vi "Get PDOMapping.vi"(8 "error in (no error)":errorcluster, 11 "OD Entry in":refnum<class "OD Entry.lvclass">) -> (0 "error out":errorcluster, 2 "PDOMapping":bool, 3 "OD Entry out":refnum<class "OD Entry.lvclass">)   [LabVIEW 2024, in "OD Entry.lvclass"]
uses:
  OD Entry.lvclass
  OD Entry.lvclass/OD Entry.ctl
  PDO Mapping Type.ctl
  EDS.lvlib
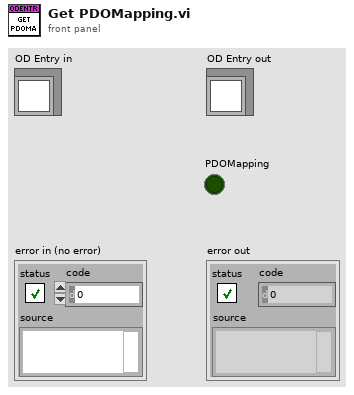
[diagram p1: front panel]
types:
  T1 = typedef "EDS.lvlib/PDO Mapping Type.ctl" = enum16{"NO", "OPTIONAL", "RPDO", "TPDO", "@DEFAULT"}
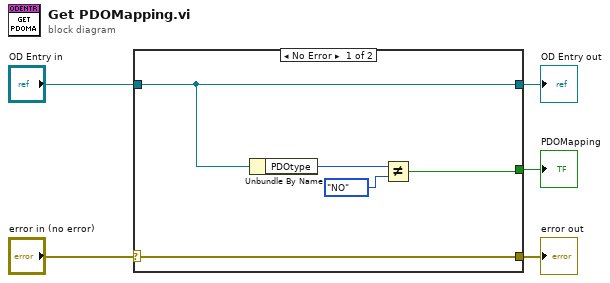
[diagram p0: block diagram]
diagram:
  n1 = case shown="No Error" "error in (no error)" {
    selector: "error in (no error)" -> [w10 w11]
    tunnel: [w10 w11] -> w4
    tunnel: [w6 w12] -> w2
    tunnel: "OD Entry in" -> [w6 w12]
    tunnel: [w7 _] -> w1
    frame No Error {
      n2 = Unbundle By Name(w6) -> ("PDOtype"=w9:T1)
      n3 = Not Equal?(x=w9, y=PDO_Mapping_Type."NO" ("PDO Mapping Type")) -> (x != y?=w7:bool)
    }
    frame Error {
    }
  }
  "error out" <- w4
  "OD Entry out" <- w2
  "PDOMapping" <- w1
